vi "wavelengthToPixel.vi"(8 "w":i32) -> (1 "r2":i32, 2 "r1":i32)   [LabVIEW 2012]
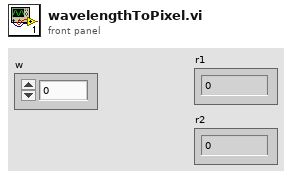
[diagram p1: front panel]
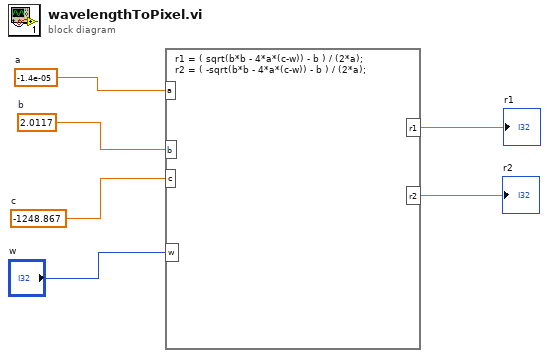
[diagram p0: block diagram]
diagram:
  w4 = -1248.867  # c
  w3 = 2.0117  # b
  w2 = -1.4e-05  # a
  n1 = formula code="r1 = ( sqrt(b*b - 4*a*(c-w)) - b ) / (2*a);\nr2 = ( -sqrt(b*b - 4*a*(c-w)) - b ) / (2*a);"("w"="w", "a"=w2, "b"=w3, "c"=w4) -> ("r2"=→"r2":dbl, "r1"=→"r1":dbl)
